vi "CLD 5 Parse Config Data File-Solution.vi"(8 "error in (no error)":errorcluster, 10 "Array In":T1[][](array[typedef])=[[{"Numeric"=1.25, "Boolean"=FALSE, "String"="One"}, {"Numeric"=1.35, "Boolean"=TRUE, "String"="Two"}, {"Numeric"=1.5, "Boolean"=FALSE, "String"="Three"}, {"Numeric"=1.0, "Boolean"=TRUE, "String"="Four"}], [{"Numeric"=2.0, "Boolean"=TRUE, "String"="Five"}, {"Numeric"=0.75, "Boolean"=FALSE, "String"="Six"}, {"Numeric"=0.9, "Boolean"=TRUE, "String"="Seven"}, {"Numeric"=0.76, "Boolean"=FALSE, "String"="Eight"}]], 11 "Get/Set":enum16{"Get", "Set"}(ring)) -> (0 "error out":errorcluster, 3 "Array Out":T1[][](array[typedef]))   [LabVIEW 2020]
doc: "CLD 5 exercise"
uses:
  CLD 5 Data Cluster.ctl
  <vilib>/Utility/config.llb/Read Key (I32).vi
  <vilib>/Utility/config.llb/Read Key (Boolean).vi
  <vilib>/Utility/config.llb/Read Key (String).vi
  <vilib>/Utility/config.llb/Read Key (Double).vi
  <vilib>/Utility/config.llb/Write Key (I32).vi
  <vilib>/Utility/config.llb/Write Key (Boolean).vi
  <vilib>/Utility/config.llb/Write Key (String).vi
  <vilib>/Utility/config.llb/Write Key (Double).vi
  <vilib>/Utility/config.llb/NI_LVConfig.lvlib
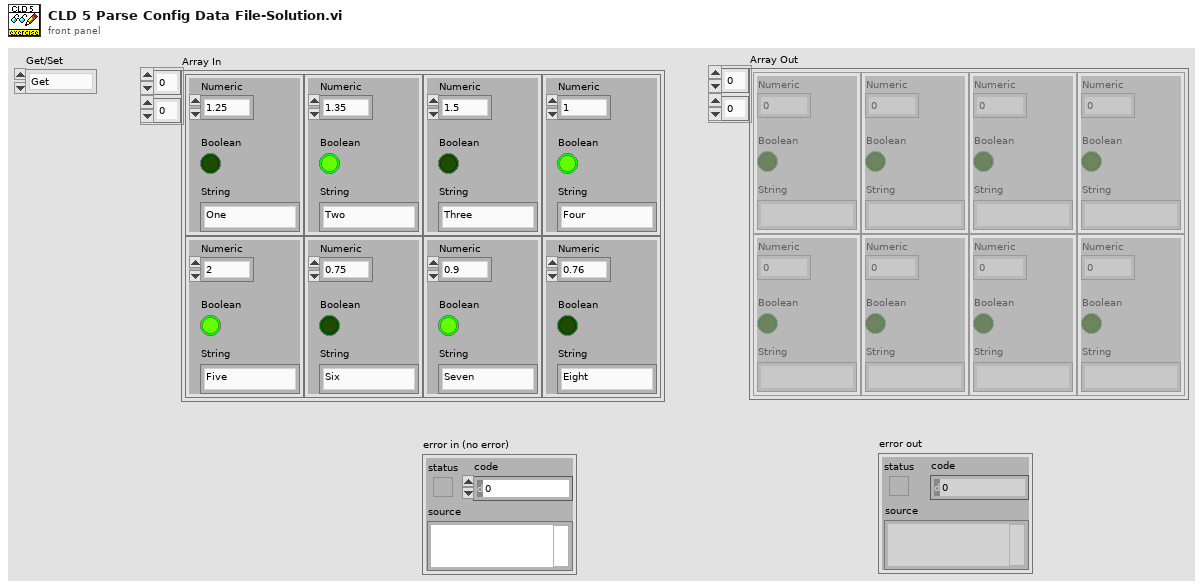
[diagram p1: front panel]
types:
  T1 = typedef "CLD 5 Data Cluster.ctl" = cluster{"Numeric":dbl, "Boolean":bool, "String":string}
  T2 = typedef "NI_LVConfig.lvlib/Config Data RefNum.ctl" = refnum<k1>
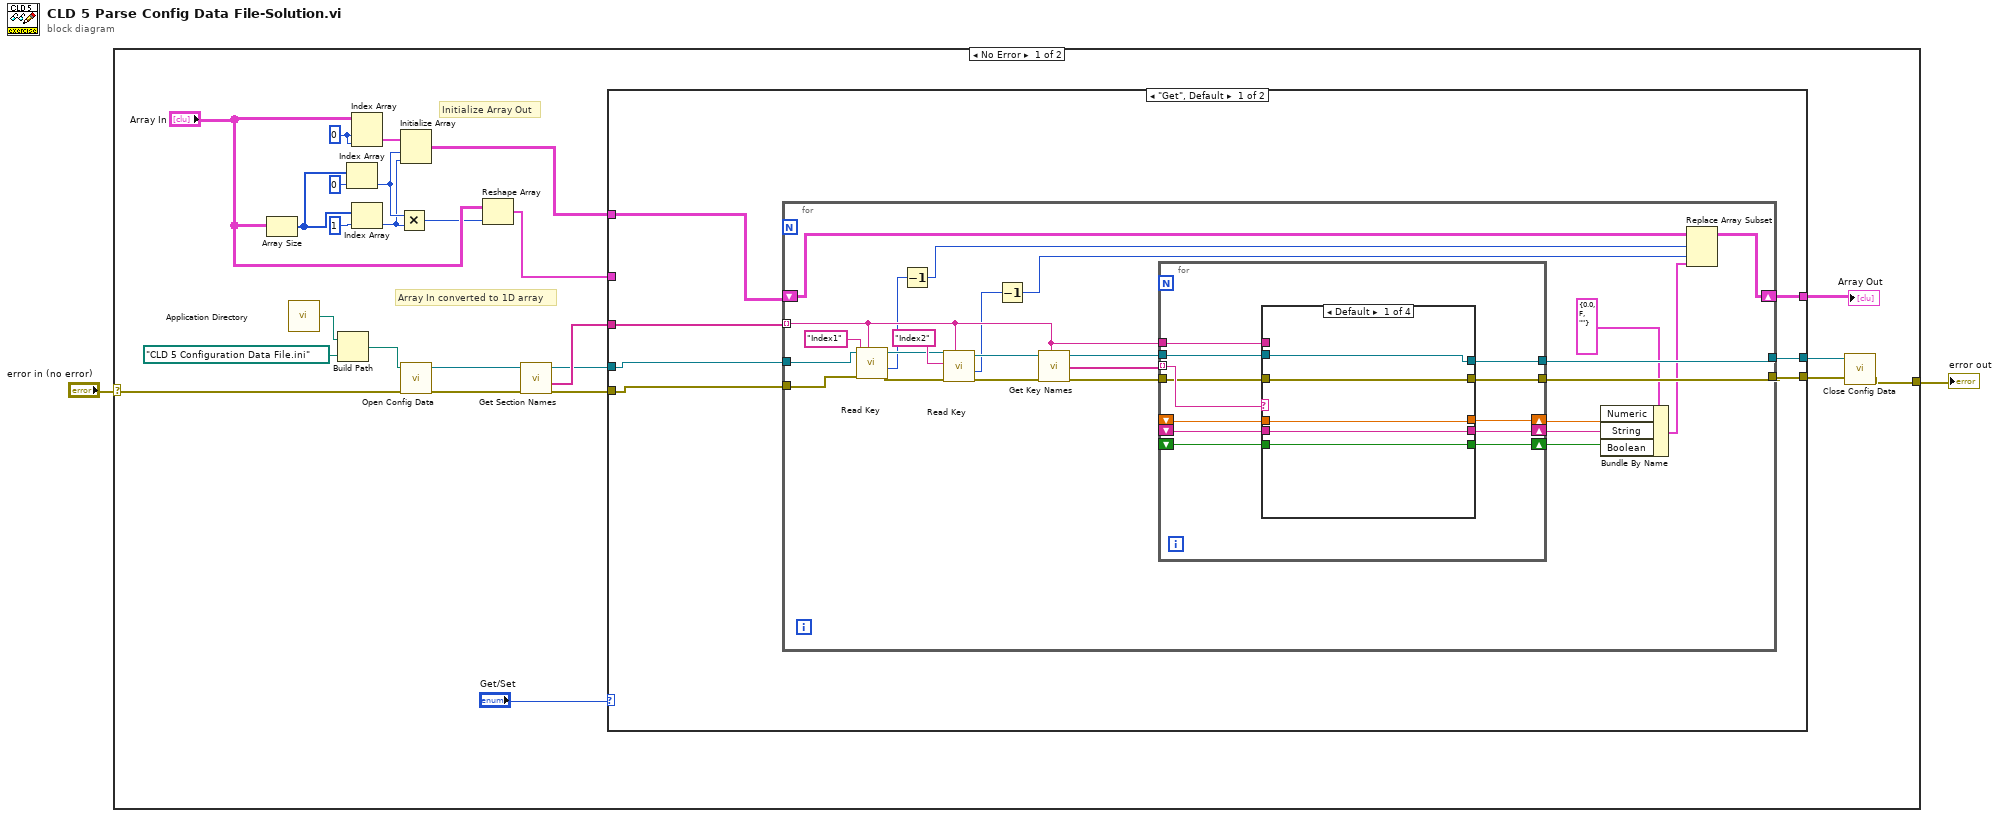
[diagram p0: block diagram]
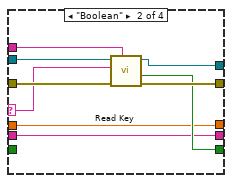
[diagram p2: hidden frame]
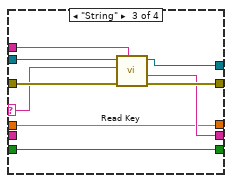
[diagram p3: hidden frame]
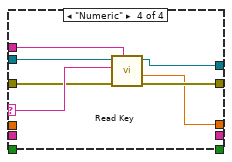
[diagram p4: hidden frame]
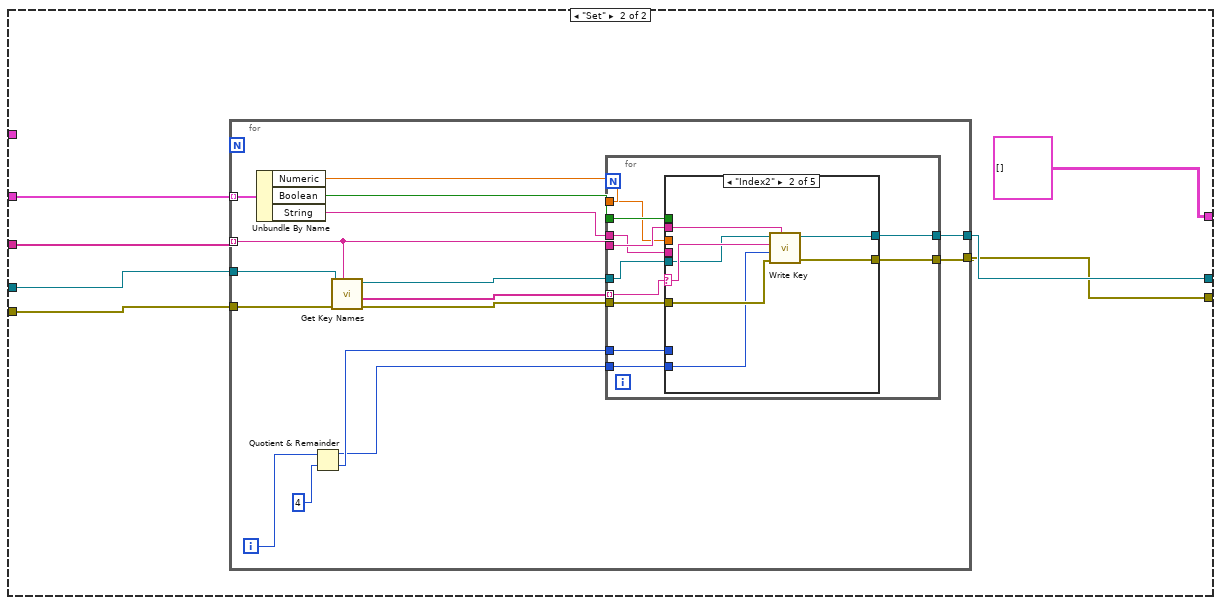
[diagram p5: hidden frame]
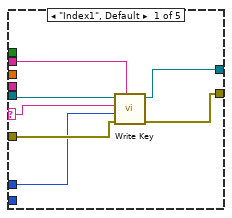
[diagram p6: hidden frame]
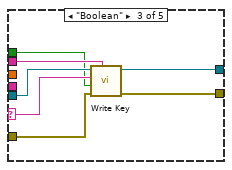
[diagram p7: hidden frame]
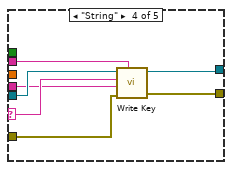
[diagram p8: hidden frame]
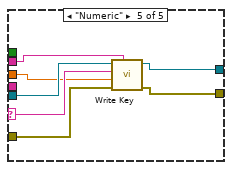
[diagram p9: hidden frame]
diagram:
  n1 = case shown="No Error" "error in (no error)" {
    selector: "error in (no error)" -> [w7 w171]
    tunnel: [w3 w171] -> w1
    frame No Error {
      w26 = 0 ("index (row)")
      # "Initialize Array Out"
      # "Array In converted to 1D array"
      n2 = Array Size(array="Array In") -> (size(s)=w24:i32[])
      n3 = call <vilib>:"Application Directory.vi"() -> ("Application Directory"=w11:path)
      n4 = Build Path(base path=w11, name or relative path=path "CLD 5 Configuration Data File.ini") -> (appended path=w12:path)
      n5 = Index Array(array=w24, index=0) -> (element=w15:i32)
      n6 = Index Array(array="Array In", index (row)=w26, index (col)=w26) -> (element=w25:T1)
      n7 = Index Array(array=w24, index=1) -> (element=w14:i32)
      n8 = Multiply(x=w15, y=w14) -> (x*y=w6:i32)
      n9 = Initialize Array(w25, w15, w14) -> (w21:T1[][])
      n10 = call <vilib>:"Open Config Data.vi"("error in (no error)"=w7, "configuration file path"=w12) -> ("error out"=w9:errorcluster, "refnum"=w8:T2)  [unwired: 7 in, 1 out]
      n11 = Reshape Array("Array In", w6) -> (w5:T1[])
      n12 = call <vilib>:"Get Section Names.vi"("error in (no error)"=w9, "refnum"=w8) -> ("error out"=w20:errorcluster, "section names"=w19:string[], "refnum out"=w18:T2)  [unwired: 7 in]
      n13 = case shown="\"Get\", Default" "Get/Set" {
        tunnel: [w33 w104] -> w4
        tunnel: [w34 w103] -> w17
        tunnel: [w32 T1[][] []] -> w13
        tunnel: w21 -> [w31 _]
        tunnel: w20 -> [w30 w106]
        tunnel: w19 -> [w29 w108]
        tunnel: w18 -> [w28 w107]
        tunnel: w5 -> [_ w102]
        frame "Get", Default {
          n14 = for {
            tunnel: w29 -> [w48] mode=indexing
            tunnel: [w50] -> w34
            tunnel: [w49] -> w33
            shift-right: [w45] -> w32
            shift-left: w31 -> [w46]
            tunnel: w30 -> [w37]
            tunnel: w28 -> [w36]
            n15 = call-poly <vilib>:"Read Key.vi"("section"=w48, "error in (no error)"=w37, "key"="Index1", "refnum"=w36) -> ("error out"=w54:errorcluster, "value"=w38:i32, "refnum out"=w57:T2)  [unwired: 4 in, 1 out]
            n16 = Decrement(x=w38) -> (x-1=w40:i32)
            n17 = call-poly <vilib>:"Read Key.vi"("section"=w48, "error in (no error)"=w54, "key"="Index2", "refnum"=w57) -> ("error out"=w55:errorcluster, "value"=w42:i32, "refnum out"=w56:T2)  [unwired: 4 in, 1 out]
            n18 = Decrement(x=w42) -> (x-1=w41:i32)
            n19 = call <vilib>:"Get Key Names.vi"("section"=w48, "error in (no error)"=w55, "refnum"=w56) -> ("error out"=w51:errorcluster, "key names"=w53:string[], "refnum out"=w52:T2)  [unwired: 5 in, 1 out]
            n20 = for {
              tunnel: w53 -> [w71] mode=indexing
              tunnel: w48 -> [w69]
              tunnel: w52 -> [w70]
              tunnel: w51 -> [w68]
              tunnel: [w67] -> w50
              tunnel: [w66] -> w49
              shift-right: [w65] -> w39
              shift-left: _ -> [w62]
              shift-right: [w64] -> w44
              shift-left: _ -> [w61]
              shift-right: [w63] -> w43
              shift-left: _ -> [w60]
              n21 = case shown="Default" w71 {
                selector: w71 -> [_ w80 w89 w99]
                tunnel: w70 -> [w72 w84 w90 w101]
                tunnel: w69 -> [_ w85 w91 w100]
                tunnel: [w72 w83 w94 w96] -> w66
                tunnel: w68 -> [w73 w82 w92 w98]
                tunnel: [w73 w81 w93 w97] -> w67
                tunnel: [w75 w77 w88 _] -> w64
                tunnel: [w76 w78 w87 w95] -> w65
                tunnel: [w74 w79 w86 _] -> w63
                tunnel: w62 -> [w76 w78 w87 _]
                tunnel: w61 -> [w75 w77 _ _]
                tunnel: w60 -> [w74 _ w86 _]
                frame Default {
                }
                frame "Boolean" {
                  n22 = call-poly <vilib>:"Read Key.vi"("section"=w85, "error in (no error)"=w82, "key"=w80, "refnum"=w84) -> ("error out"=w81:errorcluster, "value"=w79:bool, "refnum out"=w83:T2)  [unwired: 4 in, 1 out]
                }
                frame "String" {
                  n23 = call-poly <vilib>:"Read Key.vi"("section"=w91, "error in (no error)"=w92, "key"=w89, "refnum"=w90) -> ("error out"=w93:errorcluster, "value"=w88:string, "refnum out"=w94:T2)  [unwired: 4 in, 1 out]
                }
                frame "Numeric" {
                  n24 = call-poly <vilib>:"Read Key.vi"("section"=w100, "error in (no error)"=w98, "key"=w99, "refnum"=w101) -> ("error out"=w97:errorcluster, "value"=w95:dbl, "refnum out"=w96:T2)  [unwired: 4 in, 1 out]
                }
              }
            }
            n25 = Bundle By Name(cluster=T1 {"Numeric"=0.0, "Boolean"=FALSE, "String"=""} ("Cluster"), "Numeric"=w39, "String"=w44, "Boolean"=w43) -> (w47:T1)
            n26 = Replace Array Subset(array=w46, new element=w47, index (row)=w40, index (col)=w41) -> (w45:T1[][])
          }
        }
        frame "Set" {
          n27 = for {
            tunnel: w108 -> [w116] mode=indexing
            tunnel: w106 -> [w122]
            tunnel: w107 -> [w123]
            tunnel: w102 -> [w124] mode=indexing
            tunnel: [w118] -> w104
            tunnel: [w117] -> w103
            i -> [w112]
            n28 = Unbundle By Name(w124) -> ("Numeric"=w115:dbl, "Boolean"=w114:bool, "String"=w113:string)
            n29 = Quotient & Remainder(x=w112, y=4) -> (x-y*floor(x/y)=w109:i32, floor(x/y)=w110:i32)
            n30 = call <vilib>:"Get Key Names.vi"("section"=w116, "error in (no error)"=w122, "refnum"=w123) -> ("error out"=w120:errorcluster, "key names"=w119:string[], "refnum out"=w121:T2)  [unwired: 5 in, 1 out]
            n31 = for {
              tunnel: w121 -> [w135]
              tunnel: w120 -> [w133]
              tunnel: w119 -> [w127] mode=indexing
              tunnel: w116 -> [w134]
              tunnel: w115 -> [w130]
              tunnel: w114 -> [w132]
              tunnel: w113 -> [w131]
              tunnel: [w129] -> w118
              tunnel: [w128] -> w117
              tunnel: w110 -> [w126]
              tunnel: w109 -> [w125]
              n32 = case shown="\"Index2\"" w127 {
                selector: w127 -> [w142 w146 w152 w161 w170]
                tunnel: [w140 w149 w156 w163 w168] -> w129
                tunnel: [w139 w148 w155 w162 w169] -> w128
                tunnel: w135 -> [w141 w145 w154 w159 w167]
                tunnel: w134 -> [w137 w144 w153 w160 w164]
                tunnel: w133 -> [w138 w147 w151 w158 w165]
                tunnel: w132 -> [_ _ w150 _ _]
                tunnel: w131 -> [_ _ _ w157 _]
                tunnel: w130 -> [_ _ _ _ w166]
                tunnel: w126 -> [w136 _ _ _ _]
                tunnel: w125 -> [_ w143 _ _ _]
                frame "Index1", Default {
                  n33 = call-poly <vilib>:"Write Key.vi"("section"=w137, "error in (no error)"=w138, "value"=w136, "key"=w142, "refnum"=w141) -> ("error out"=w139:errorcluster, "refnum out"=w140:T2)  [unwired: 4 in, 1 out]
                }
                frame "Index2" {
                  n34 = call-poly <vilib>:"Write Key.vi"("section"=w144, "error in (no error)"=w147, "value"=w143, "key"=w146, "refnum"=w145) -> ("error out"=w148:errorcluster, "refnum out"=w149:T2)  [unwired: 4 in, 1 out]
                }
                frame "Boolean" {
                  n35 = call-poly <vilib>:"Write Key.vi"("section"=w153, "error in (no error)"=w151, "value"=w150, "key"=w152, "refnum"=w154) -> ("error out"=w155:errorcluster, "refnum out"=w156:T2)  [unwired: 4 in, 1 out]
                }
                frame "String" {
                  n36 = call-poly <vilib>:"Write Key.vi"("section"=w160, "error in (no error)"=w158, "value"=w157, "key"=w161, "refnum"=w159) -> ("error out"=w162:errorcluster, "refnum out"=w163:T2)  [unwired: 4 in, 1 out]
                }
                frame "Numeric" {
                  n37 = call-poly <vilib>:"Write Key.vi"("section"=w164, "error in (no error)"=w165, "value"=w166, "key"=w170, "refnum"=w167) -> ("error out"=w169:errorcluster, "refnum out"=w168:T2)  [unwired: 4 in, 1 out]
                }
              }
            }
          }
        }
      }
      "Array Out" <- w13
      n38 = call <vilib>:"Close Config Data.vi"("error in (no error)"=w17, "refnum"=w4) -> ("error out"=w3:errorcluster)  [unwired: 8 in, 1 out]
    }
    frame Error {
    }
  }
  "error out" <- w1
